vi "Set Next Address.vi"(6 "physical":i32, 7 "length":i32, 9 "highAdd":i32, 10 "lowAdd":i32, 11 "data":i32) -> (2 "function return":u32, 3 "data out":i32)   [LabVIEW 2018, in "Copy of Andor SDK.lvlib"]
doc: "EXPNETTYPE unsigned int WINAPI SetNextAddress(at_32 * data, long lowAdd, long highAdd, long length, long physical);"
uses:
  Copy of Andor SDK.lvlib
  <userlib>/Andor SDK/ATMCD32D.dll
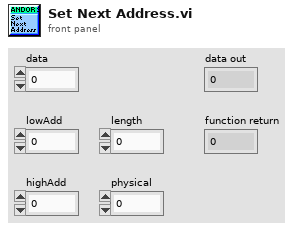
[diagram p1: front panel]
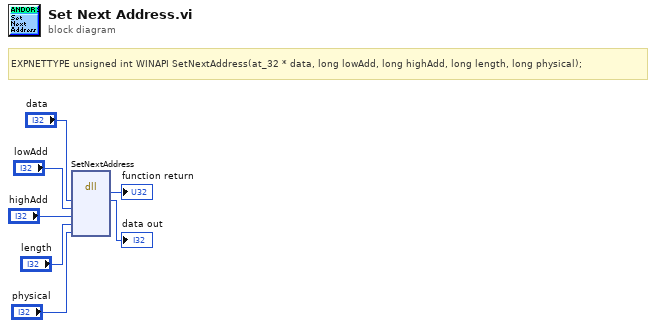
[diagram p0: block diagram]
diagram:
  # "EXPNETTYPE unsigned int WINAPI SetNextAddress(at_32 * data, long lowAdd, long highAdd, long length, long physical);"
  n1 = dll-call lib="C:/Program Files (x86)/National Instruments/LabVIEW 2018/user.lib/Andor SDK/ATMCD32D.*" fn="SetNextAddress"("data"="data", "lowAdd"="lowAdd", "highAdd"="highAdd", "length"="length", "physical"="physical") -> (→"function return":u32, "data"=→"data out":i32)  [unwired: 7 in, 2 out]
